vi "Save TestDefinition to XML.vi"(8 "error in (no error)":errorcluster, 10 "SaveDir":path, 11 "TestDefinition":T1={"Test Sequence"=[{"TTrigger"=-130.0, "Direction"=enum."Falling", "TDelay"=0.0, "Type"=enum."No Test", "Pre-Log (s)"=10.0, "Duration (s)"=30.0, "Post-Log(s)"=100.0}, {"TTrigger"=-80.0, "Direction"=enum."Rising", "TDelay"=0.0, "Type"=enum."Heater Test", "Pre-Log (s)"=10.0, "Duration (s)"=30.0, "Post-Log(s)"=100.0}, {"TTrigger"=-50.0, "Direction"=enum."Rising", "TDelay"=30.0, "Type"=enum."Actuation Test", "Pre-Log (s)"=10.0, "Duration (s)"=30.0, "Post-Log(s)"=100.0}, {"TTrigger"=-40.0, "Direction"=enum."Rising", "TDelay"=0.0, "Type"=enum."Actuation Test", "Pre-Log (s)"=10.0, "Duration (s)"=30.0, "Post-Log(s)"=100.0}, {"TTrigger"=-30.0, "Direction"=enum."Rising", "TDelay"=0.0, "Type"=enum."Actuation Test", "Pre-Log (s)"=10.0, "Duration (s)"=30.0, "Post-Log(s)"=100.0}, {"TTrigger"=-20.0, "Direction"=enum."Rising", "TDelay"=0.0, "Type"=enum."Actuation Test", "Pre-Log (s)"=10.0, "Duration (s)"=30.0, "Post-Log(s)"=100.0}, {"TTrigger"=-10.0, "Direction"=enum."Rising", "TDelay"=0.0, "Type"=enum."Actuation Test", "Pre-Log (s)"=10.0, "Duration (s)"=30.0, "Post-Log(s)"=100.0}, {"TTrigger"=0.0, "Direction"=enum."Rising", "TDelay"=0.0, "Type"=enum."Actuation Test", "Pre-Log (s)"=10.0, "Duration (s)"=30.0, "Post-Log(s)"=100.0}, {"TTrigger"=10.0, "Direction"=enum."Rising", "TDelay"=0.0, "Type"=enum."Actuation Test", "Pre-Log (s)"=10.0, "Duration (s)"=30.0, "Post-Log(s)"=100.0}, {"TTrigger"=20.0, "Direction"=enum."Rising", "TDelay"=0.0, "Type"=enum."Actuation Test", "Pre-Log (s)"=10.0, "Duration (s)"=30.0, "Post-Log(s)"=100.0}, {"TTrigger"=30.0, "Direction"=enum."Rising", "TDelay"=0.0, "Type"=enum."Actuation Test", "Pre-Log (s)"=10.0, "Duration (s)"=30.0, "Post-Log(s)"=100.0}, {"TTrigger"=40.0, "Direction"=enum."Rising", "TDelay"=0.0, "Type"=enum."Actuation Test", "Pre-Log (s)"=10.0, "Duration (s)"=30.0, "Post-Log(s)"=100.0}], "ActuationsPerLoop"=10, "Temperature Log Period(ms)"=100, "PSU  Log Period (ms)"=2, "Diode Test Options"={"Temp.Tol"=0.0, "Max IDark"=[], "Min ILight"=[], "Min TEC \nCurrent"=0.0, "Max TEC \nCurrent"=0.0}, "Heater Test Options"={"Heater Nominal Current (A)"=0.67, "Heater Current Tolerance (%)"=20.0}} {"Heater Test Options"."Heater Current Tolerance (%)" min=1.0 max=100.0; "Heater Test Options"."Heater Nominal Current (A)" min=0.0 max=1.0; "Test Sequence"."Post-Log(s)" format="%#_13g"; "Test Sequence"."Pre-Log (s)" format="%#_13g"; "Test Sequence"."Duration (s)" format="%#_13g"}) -> (0 "error out":errorcluster)   [LabVIEW 2025]
doc: "Saves the user-specified configuration data to an XML file. This is used to remember settings between executions."
uses:
  controls/TestDefinition.ctl
  controls/SingleTest.ctl
  controls/TestType.ctl
  controls/Diode Test Options.ctl
  controls/HTR Test Options.ctl
  <vilib>/Utility/xml.llb/Write to XML File(string).vi
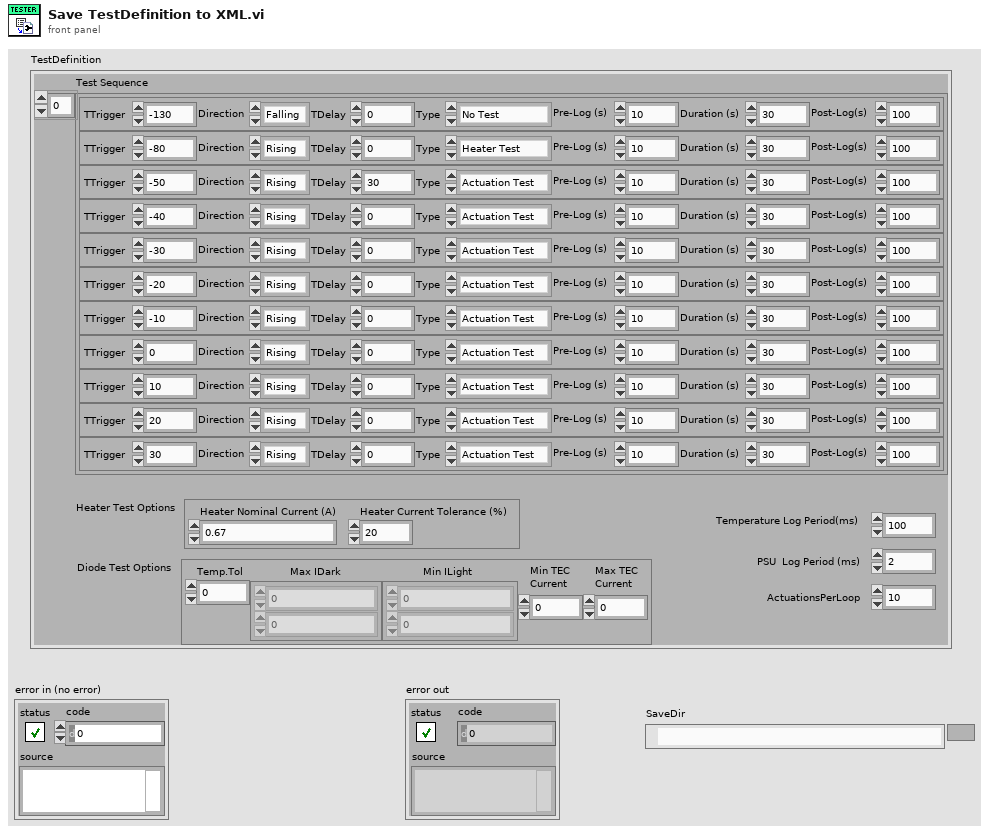
[diagram p1: front panel]
types:
  T1 = typedef "TestDefinition.ctl" = cluster{"Test Sequence":T2[], "ActuationsPerLoop":i32, "Temperature Log Period(ms)":i64, "PSU  Log Period (ms)":i64, "Diode Test Options":T4, "Heater Test Options":T5}
  T2 = typedef "SingleTest.ctl" = cluster{"TTrigger":dbl, "Direction":enum16{"Rising", "Falling"}, "TDelay":dbl, "Type":T3, "Pre-Log (s)":dbl, "Duration (s)":dbl, "Post-Log(s)":dbl}
  T3 = typedef "TestType.ctl" = enum16{"No Test", "Heater Test", "Actuation Test", "Diode Test"}
  T4 = typedef "Diode Test Options.ctl" = cluster{"Temp.Tol":dbl, "Max IDark":dbl[], "Min ILight":dbl[], "Min TEC \nCurrent":dbl, "Max TEC \nCurrent":dbl}
  T5 = typedef "HTR Test Options.ctl" = cluster{"Heater Nominal Current (A)":dbl, "Heater Current Tolerance (%)":dbl}
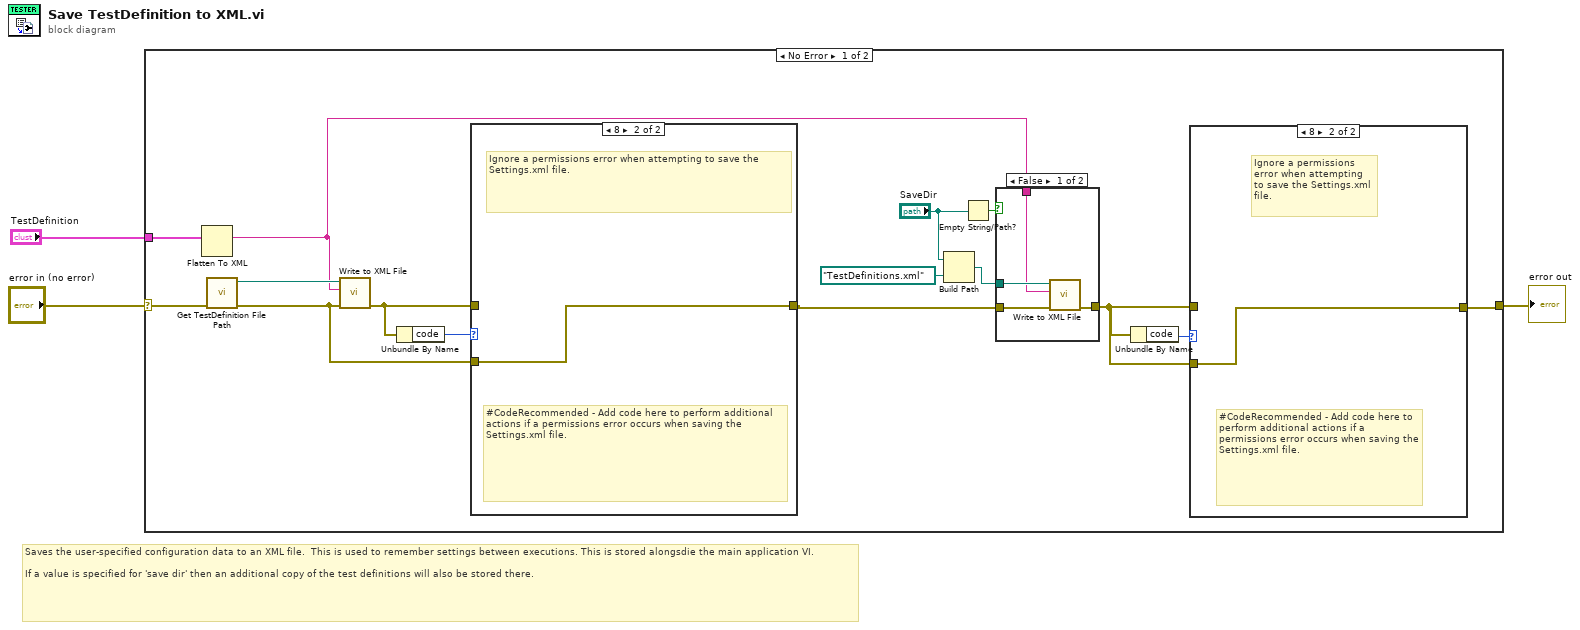
[diagram p0: block diagram]
diagram:
  # "Saves the user-specified configuration data to an XML file.  This is used to remember settings between executions. This is stored alongsdie the main application VI.\n\nIf a value is specified for 'save dir' then an additional copy of the test definitions will also be stored there."
  n1 = case shown="No Error" "error in (no error)" {
    selector: "error in (no error)" -> [w16 w28]
    tunnel: [w9 w28] -> w2
    tunnel: "TestDefinition" -> [w18 _]
    frame No Error {
      n2 = Flatten To XML(6:w18) -> (2:w10:string)
      n3 = call "Get TestDefinition File Path.vi"("error in (no error)"=w16) -> ("error out"=w13:errorcluster, "XML File Path"=w17:path)  [unwired: 9 in]
      n4 = call-poly <vilib>:"Write to XML File.vi"("error in (no error)"=w13, "XML Input"=w10, "XML File Path"=w17) -> ("error out"=w14:errorcluster)  [unwired: 6 in, 2 out]
      n5 = Unbundle By Name(w14) -> ("code"=w15:i32)
      n6 = case shown="8" w15 {
        tunnel: [w26 w27] -> w11
        tunnel: w14 -> [w26 _]
        tunnel: w13 -> [_ w27]
        frame Default {
        }
        frame 8 {
          # "Ignore a permissions error when attempting to save the Settings.xml file."
          # "#CodeRecommended - Add code here to perform additional actions if a permissions error occurs when saving the Settings.xml file."
        }
      }
      n7 = Build Path(base path="SaveDir", name or relative path=path "TestDefinitions.xml" ("string")) -> (appended path=w6:path)
      n8 = Empty String/Path?(string/path="SaveDir") -> (empty?=w12:bool)
      n9 = case shown="False" w12 {
        tunnel: [w23 w25] -> w7
        tunnel: w11 -> [w24 w25]
        tunnel: w6 -> [w22 _]
        tunnel: w10 -> [w21 _]
        frame False {
          n10 = call-poly <vilib>:"Write to XML File.vi"("error in (no error)"=w24, "XML Input"=w21, "XML File Path"=w22) -> ("error out"=w23:errorcluster)  [unwired: 6 in, 2 out]
        }
        frame True {
        }
      }
      n11 = Unbundle By Name(w7) -> ("code"=w8:i32)
      n12 = case shown="8" w8 {
        tunnel: [w19 w20] -> w9
        tunnel: w7 -> [_ w20]
        tunnel: w7 -> [w19 _]
        frame Default {
        }
        frame 8 {
          # "Ignore a permissions error when attempting to save the Settings.xml file."
          # "#CodeRecommended - Add code here to perform additional actions if a permissions error occurs when saving the Settings.xml file."
        }
      }
    }
    frame Error {
    }
  }
  "error out" <- w2
